vi "CAN Loopback.vi"() -> ()   [LabVIEW 2020]
doc: "This example demonstrates basic communication on the CAN bus. The example runs standalone (without a host VI).\n\nIt reads CAN frames on CAN 0 and displays a count along with the most recent frame. It transmits a CAN frame on CAN 1 each time you select the Transmit button. You can use the example simply by connecting a CAN cable (powered) between CAN 0 and CAN 1. To use the example with an external CAN device (such as an ECU), connect the device to CAN 0, then change the CAN Output node from CAN 1 to CAN 0. This enables you to interactively transmit and receive CAN frames with the external device.\n\nThis example assumes the following configuration for CAN 0 and CAN 1: Auto Start = True, Listen Only = False, Input Timeout = 10000ms, Output Timeout = 10000ms. The CAN Input and CAN Output nodes are configured to use Cluster for the CAN frame. For more information on configuration, refer to the Help for the NI 9852/9853 CAN module.\n\nIf you change this example such that the loops exit normally (such as a stop button), you must add the CAN Stop method to stop CAN communication before the VI stops execution. Only the LabVIEW abort button stops CAN communication when running standalone (no host VI).\n\nNote: Prior to running the VI, you will need to specify the VISA resource name for the FPGA target. You can specify the VISA resource name by right clicking the FPGA Target in the Project Explorer, then selecting Properties... and then specifying the VISA resource string."
uses:
  <vilib>/eio/EIONode/EIONode.xnode
  Instance           1 24Saved   CAN Basic (FPGA) .vi
  <vilib>/rvi/eio/common/nirviEmuTemplateMethod_errors.vi
  <vilib>/LabVIEW Targets/FPGA/RIO/nicrio_985x_controls.llb/CAN_IO_Frame Type.ctl
  <vilib>/LabVIEW Targets/FPGA/RIO/nicrio_985x_controls.llb/CAN_IO_Frame Cluster.ctl
panel:
  in  "Transmit Frame":T1={"timestamp high"=0, "timestamp low"=0, "identifier"=5, "type"=enum."Data Frame", "info A"=0, "info B"=0, "data length"=8, "data"=[1, 2, 3, 4, 5, 6, 7, 8]} {"identifier" format="%x"; "timestamp high" format="%08x"; "timestamp low" format="%08x"; "data" format="%.0x"}
  out "Recent Receive":T1={"timestamp high"=0, "timestamp low"=0, "identifier"=0, "type"=enum."Data Frame", "info A"=0, "info B"=0, "data length"=0, "data"=[0, 0, 0, 0, 0, 0, 0, 0]} {"identifier" format="%x"; "timestamp high" format="%08x"; "timestamp low" format="%08x"; "data" format="%.0x"}
  in  "Transmit":bool
  out "Total Received":u32 format="%.0x"
  # "See VI Info <Ctrl+I> for more information on how to use this example"
  # "Note: Use the LabVIEW Abort Execution button \n(Stop sign) to stop the VI."
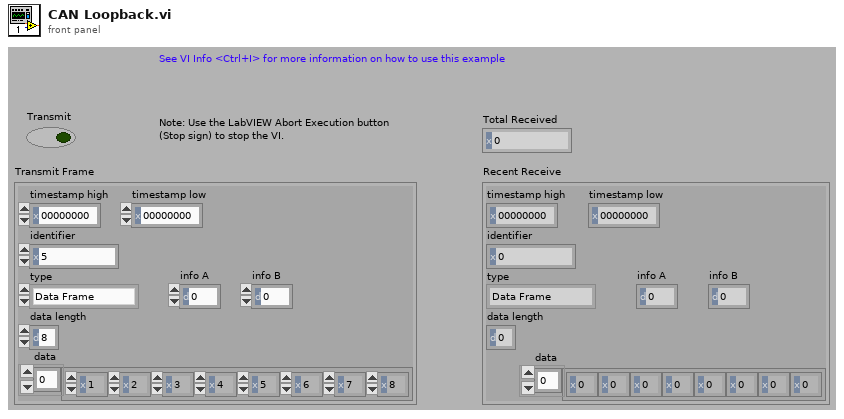
[diagram p1: front panel]
types:
  T1 = typedef "CAN_IO_Frame Cluster.ctl" = cluster{"timestamp high":u32, "timestamp low":u32, "identifier":u32, "type":T2, "info A":u8, "info B":u8, "data length":u8, "data":u8[]}
  T2 = typedef "CAN_IO_Frame Type.ctl" = enum8{"Data Frame", "Remote Frame", "(reserved)", "(reserved) ", "(reserved)  ", "(reserved)   ", "Bus Error", "Transceiver Fault"}
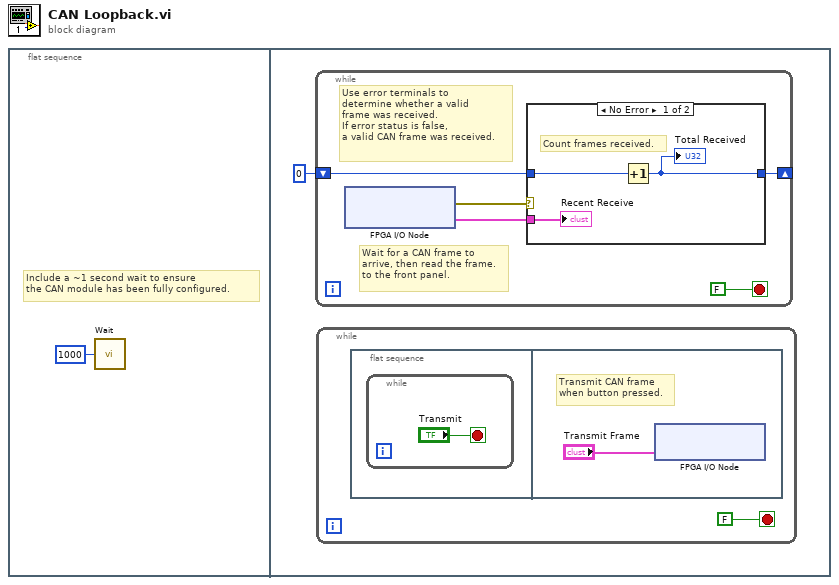
[diagram p0: block diagram]
diagram:
  n1 = flat-sequence {
    frame #0 {
      # "Include a ~1 second wait to ensure \nthe CAN module has been fully configured."
      n2 = call "Wait"("Count(mSec)"=u16 1000) -> ()  [unwired: 1 out]
    }
    frame #1 {
      n3 = while {
        shift-right: [w9] -> _
        shift-left: u32 0 ("Total Received") -> [w10]
        stop <- FALSE stop-if-true
        # "Use error terminals to \ndetermine whether a valid\nframe was received.  \nIf error status is false, \na valid CAN frame was received."
        # "Wait for a CAN frame to\narrive, then read the frame. \nto the front panel."
        n4 = xnode "FPGA I/O Node"() -> ("error out"=w6:errorcluster, "Mod8/CAN0"=w7:T1)  [unwired: 2 in, 1 out]
        n5 = case shown="No Error" w6 {
          tunnel: w7 -> [w11 _]
          tunnel: w10 -> [w13 w14]
          tunnel: [w12 w14] -> w9
          frame No Error {
            # "Count frames received."
            n6 = Increment(x=w13) -> (x+1=w12:u32)
            "Total Received" <- w12
            "Recent Receive" <- w11
          }
          frame Error {
          }
        }
      }
      n7 = while {
        stop <- FALSE stop-if-true
        n8 = flat-sequence {
          frame #0 {
            n9 = while {
              stop <- "Transmit" stop-if-true
            }
          }
          frame #1 {
            # "Transmit CAN frame \nwhen button pressed."
            n10 = xnode "FPGA I/O Node"("Mod8/CAN1"="Transmit Frame") -> ()  [unwired: 1 in, 1 out]
          }
        }
      }
    }
  }
